vi "sv_Demodulation with Decimation.vi"(0 "x[n]":dbl[][](array[numeric]) format="%.2f", 1 "reset? (True)":bool=TRUE, 2 "zero delay? (F)":bool, 5 "fs":dbl=1.0 format="%.2f", 9 "fc [Hz]":dbl[](array[numeric])=[0.0] format="%.2f", 11 "decimation factor":i32=16, 12 "stop band attenuation":u16(ring) items=["72 dB", "96 dB", "120 dB"], 14 "phase setting":T1) -> (3 "lags":i32, 4 "magnitudes (RMS)":dbl[][][](array[numeric]) format="%.2f", 6 "phase lag":dbl[][][](array[numeric]) format="%.2f", 10 "new fs [Hz]":dbl format="%.2f", 15 "error out":errorcluster)   [LabVIEW 2017, in "SoundVib_ContSweptSine.lvlib"]
uses:
  <vilib>/addons/Sound and Vibration/svt_Continuous Swept Sine/SoundVib_ContSweptSine.lvlib
  <vilib>/addons/Sound and Vibration/Order Analysis/Misc/OAT Convert Phase (N Channels).vi
  <vilib>/Analysis/NI_AALPro.lvlib
  <vilib>/addons/Sound and Vibration/Order Analysis/Resample Order Tracking/SoundVib_Resampling.lvlib
panel:
  # "Demodulation"
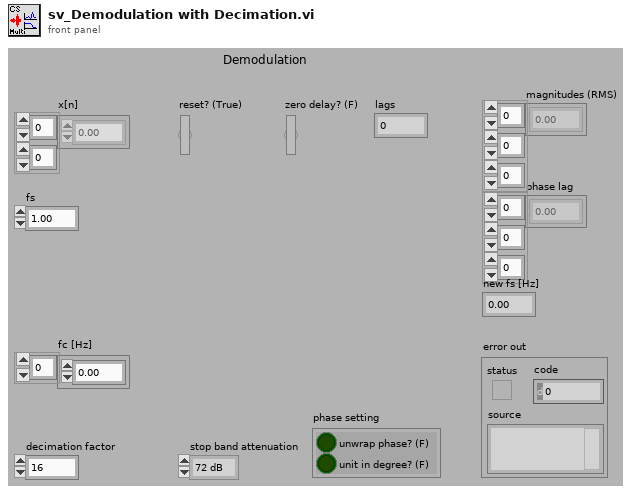
[diagram p1: front panel]
types:
  T1 = cluster{"unwrap phase? (F)":bool, "unit in degree? (F)":bool}
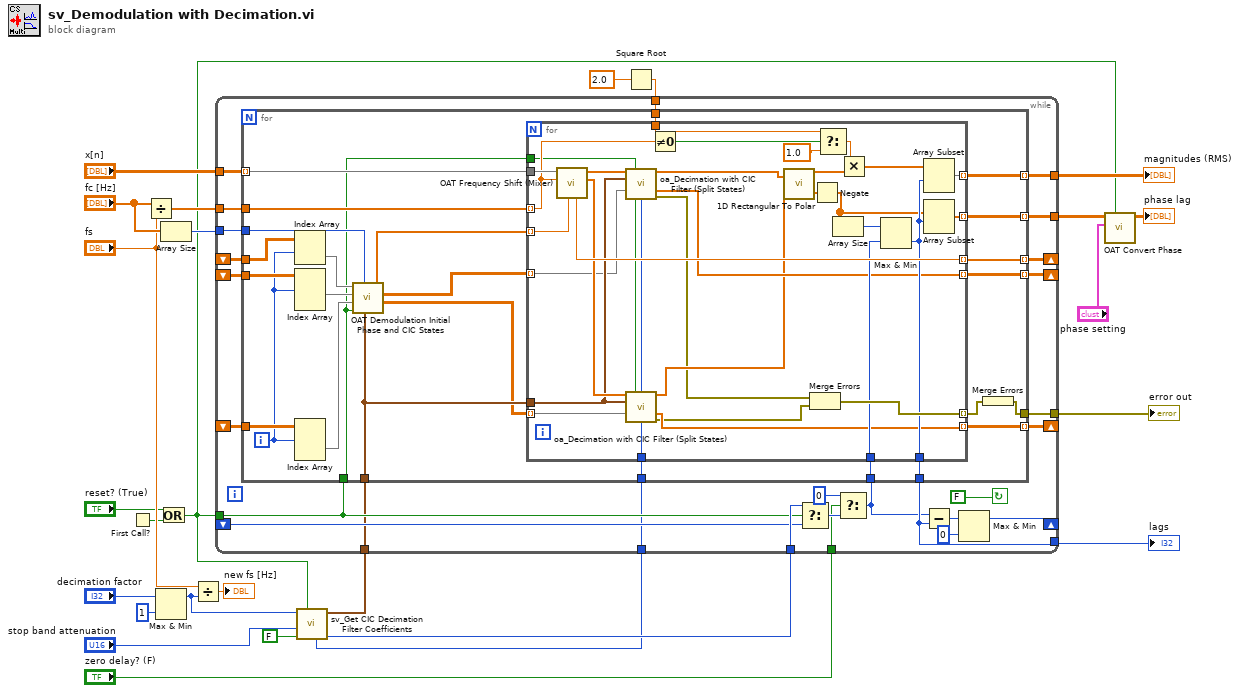
[diagram p0: block diagram]
diagram:
  n1 = First Call?() -> (First Call?: T/F=w15:bool)
  n2 = Divide(x="fc [Hz]", y="fs") -> (x/y=w26:dbl[])
  n3 = Max & Min(x="decimation factor", y=1) -> (max(x,y)=w2:i32)  [unwired: 1 out]
  n4 = Or(x="reset? (True)", y=w15) -> (x .or. y?=w7:bool)
  n5 = Array Size(array="fc [Hz]") -> (size(s)=w25:i32)
  n6 = Divide(x="fs", y=w2) -> (x/y=→"new fs [Hz]":dbl)
  n7 = call <vilib>:"sv_Get CIC Decimation Filter Coefficients.vi"("reset? (True)"=w7, "alias protect in final transition"=FALSE, "stop band attenuation"="stop band attenuation", "decimation/interpolation factor"=w2) -> ("delay"=w8:i32, "CIC Settings"=w6:cluster{"Numeric":i32, i32, i32}, "interpolation factor"=w5:i32)  [unwired: 5 out]
  n8 = Square Root(x=2.0) -> (sqrt(x)=w23:dbl)
  n9 = while {
    tunnel: w23 -> [w47]
    tunnel: w25 -> [w48]
    shift-left: _ -> [w49]
    shift-right: [w50] -> _
    tunnel: w7 -> [w42]
    tunnel: w26 -> [w52]
    tunnel: "x[n]" -> [w53]
    tunnel: [w46] -> w10
    tunnel: [w45] -> w22
    tunnel: [w44] -> w13
    tunnel: [w40] -> w12
    shift-right: [w37] -> _
    shift-left: _ -> [w41]
    tunnel: w8 -> [w43]
    tunnel: w6 -> [w36]
    tunnel: w5 -> [w35]
    tunnel: "zero delay? (F)" -> [w31]
    shift-right: [w30] -> _
    shift-left: _ -> [w29]
    shift-right: [w28] -> _
    shift-left: _ -> [w27]
    stop <- FALSE continue-if-true
    n10 = Select(t=w43, s=w42, f=w41) -> (s? t:f=w33:i32)
    n11 = Select(t=0 ("x"), s=w31, f=w33) -> (s? t:f=w32:i32)
    n12 = for {
      tunnel: w53 -> [w79] mode=indexing
      tunnel: w52 -> [w78]
      tunnel: [w77] -> w50 mode=indexing
      tunnel: w49 -> [w68]
      tunnel: w48 -> [w56]
      tunnel: w47 -> [w75]
      tunnel: [w74] -> w46 mode=indexing
      tunnel: [w73] -> w45 mode=indexing
      tunnel: [w71] -> w44
      tunnel: w42 -> [w55]
      tunnel: w32 -> [w70]
      tunnel: [w69] -> w40
      tunnel: w36 -> [w67]
      tunnel: w35 -> [w66]
      tunnel: [w63] -> w30 mode=indexing
      tunnel: w29 -> [w62]
      tunnel: [w60] -> w28 mode=indexing
      tunnel: w27 -> [w59]
      i -> [w54]
      n13 = Index Array(array=w68, index (row)=w54) -> (element=w65:dbl[])  [unwired: 1 in]
      n14 = Index Array(array=w62, index (dim 0)=w54) -> (element=w61:dbl[][])  [unwired: 2 in]
      n15 = Index Array(array=w59, index (dim 0)=w54) -> (element=w58:dbl[][])  [unwired: 2 in]
      n16 = call <vilib>:"OAT Demodulation Initial Phase and CIC States.vi"("CIC filter settings"=w67, "num of orders"=w56, "reset? (True)"=w55, "CIC Image in"=w58, "CIC Real in"=w61, "start phase in"=w65) -> ("CIC Image"=w57:dbl[][], "CIC Real"=w64:dbl[][], "start phase out"=w76:dbl[])  [unwired: 3 in]
      n17 = for {
        tunnel: w79 -> [w108]
        tunnel: w78 -> [w97] mode=indexing
        tunnel: [w110] -> w77 mode=indexing
        tunnel: w76 -> [w88] mode=indexing
        tunnel: w75 -> [w95]
        tunnel: [w101] -> w74 mode=indexing
        tunnel: [w102] -> w73 mode=indexing
        tunnel: [w104] -> w72 mode=indexing
        tunnel: w70 -> [w99]
        tunnel: [w98] -> w69
        tunnel: w55 -> [w92]
        tunnel: w67 -> [w90]
        tunnel: w66 -> [w89]
        tunnel: w64 -> [w87] mode=indexing
        tunnel: [w86] -> w63 mode=indexing
        tunnel: w57 -> [w85] mode=indexing
        tunnel: [w84] -> w60 mode=indexing
        n18 = call <vilib>:"OAT Frequency Shift (Mixer).vi"("initial phase"=w88, "fc"=w97, "X"=w108) -> ("imaginary"=w107:dbl[], "real"=w106:dbl[], "final phase"=w110:dbl)  [unwired: 6 out]
        n19 = call <vilib>:"oa_Decimation with CIC Filter (Split States).vi"("x[n]"=w106, "reset? (True)"=w92, "CIC decimation setting"=w90, "CIC state"=w87, "interpolation factor"=w89) -> ("x[n] out"=w82:dbl[], "final CIC state"=w86:dbl[], "error out"=w80:errorcluster)  [unwired: 3 in, 5 out]
        n20 = call <vilib>:"oa_Decimation with CIC Filter (Split States).vi"("x[n]"=w107, "reset? (True)"=w92, "CIC decimation setting"=w90, "CIC state"=w85, "interpolation factor"=w89) -> ("x[n] out"=w83:dbl[], "final CIC state"=w84:dbl[], "error out"=w81:errorcluster)  [unwired: 3 in, 5 out]
        n21 = Not Equal To 0?(x=w97) -> (x != 0?=w96:bool)
        n22 = call <vilib>:"1D Rectangular To Polar.vi"("X"=w82, "Y"=w83) -> ("Magnitude"=w109:dbl[], "Phase"=w105:dbl[])  [unwired: 1 out]
        n23 = Merge Errors(w80, w81) -> (w104:errorcluster)
        n24 = Negate(x=w105) -> (-x=w91:dbl[])
        n25 = Select(t=w95, s=w96, f=1.0) -> (s? t:f=w94:dbl)
        n26 = Array Size(array=w91) -> (size(s)=w100:i32)
        n27 = Multiply(x=w94, y=w109) -> (x*y=w103:dbl[])
        n28 = Max & Min(x=w100, y=w99) -> (min(x,y)=w98:i32)  [unwired: 1 out]
        n29 = Array Subset(array=w103, index=w98) -> (w102:dbl[])  [unwired: 1 in]
        n30 = Array Subset(array=w91, index=w98) -> (w101:dbl[])  [unwired: 1 in]
      }
      n31 = Merge Errors(w72) -> (w71:errorcluster)
    }
    n32 = Subtract(x=w32, y=w40) -> (x-y=w39:i32)
    n33 = Max & Min(x=w39, y=0) -> (max(x,y)=w37:i32)  [unwired: 1 out]
  }
  "error out" <- w13
  "magnitudes (RMS)" <- w22
  "lags" <- w12
  n34 = call-poly <vilib>:"OAT Convert Phase.vi"("reset (TRUE)"=w7, "desired phase setting"="phase setting", "phase in"=w10) -> ("phase out"=→"phase lag":dbl[][][])  [unwired: 1 in, 7 out]
